vi "Get Channel Destinations.vi"(10 "Source":string, 11 "SLSC Switch in":refnum<class "SLSC Switch.lvclass">) -> (2 "Array":string[](array[string]))   [LabVIEW 2015, in "SLSC Switch.lvlib" / "SLSC Switch.lvclass"]
uses:
  SLSC Switch.lvclass
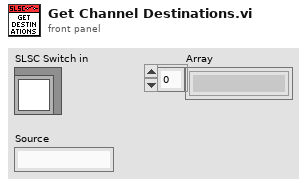
[diagram p1: front panel]
types:
  T1 = typedef "SLSC Switch.lvlib/SLSC Switch.lvclass/Connection.ctl" = cluster{"channel 1":string, "channel 2":string}
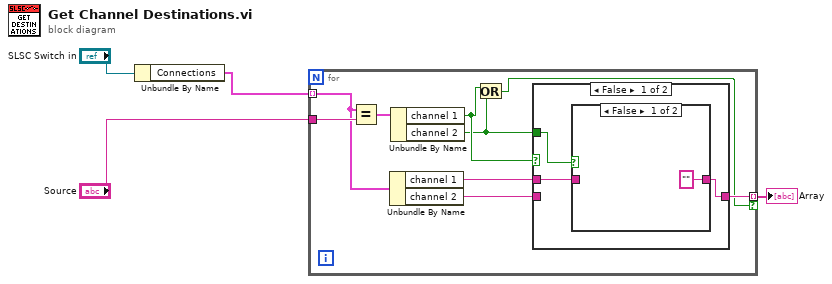
[diagram p0: block diagram]
diagram:
  n1 = Unbundle By Name("SLSC Switch in") -> ("Connections"=w2:T1[])
  n2 = for {
    tunnel: w2 -> [w11] mode=indexing
    tunnel: "Source" -> [w13]
    tunnel: [w6] -> w4 mode=indexing if=w5
    n3 = Equal?(x=w11, y=w13) -> (x = y?=w12:cluster{"channel 1":bool, "channel 2":bool})
    n4 = Unbundle By Name(w11) -> ("channel 1"=w10:string, "channel 2"=w9:string)
    n5 = Unbundle By Name(w12) -> ("channel 1"=w8:bool, "channel 2"=w7:bool)
    n6 = Or(x=w8, y=w7) -> (x .or. y?=w5:bool)
    n7 = case shown="False" w8 {
      tunnel: w10 -> [w14 _]
      tunnel: w9 -> [_ w19]
      tunnel: w7 -> [w16 _]
      tunnel: [w15 w19] -> w6
      frame False {
        n8 = case shown="False" w16 {
          tunnel: ["" ("channel 1") w18] -> w15
          tunnel: w14 -> [_ w18]
          frame False {
          }
          frame True {
          }
        }
      }
      frame True {
      }
    }
  }
  "Array" <- w4
